vi "ctet_smu_User Main.vi"() -> ()   [LabVIEW 2019, in "ctet_smu User Library.lvlib"]
uses:
  ctet_smu User Library.lvlib
  Servers/ctet_smu/ctet_smu Class/typeDefs/Server State Data.ctl
  Types/ctet_smu.ctl
  Servers/ctet_smu/ctet_smu Class/RPC Messages/measurementservice_SMUConfigResponse/measurementservice_SMUConfigResponse_Data.ctl
  Servers/ctet_smu/ctet_smu Class/RPC Messages/measurementservice_ErrorOut/measurementservice_ErrorOut_Data.ctl
  Servers/ctet_smu/ctet_smu Class/ctet_smu.lvclass/ctet_smu.ctl
  Servers/ctet_smu/ctet_smu Class/ctet_smu.lvclass
panel:
  out "error out":errorcluster
  in  "error in (no error)":errorcluster
  in  "Stop":bool
  in  "Server Address":string="0.0.0.0:50052"
  in  "Server Certificate File (.crt)":path
  in  "Server Key File (.key)":path
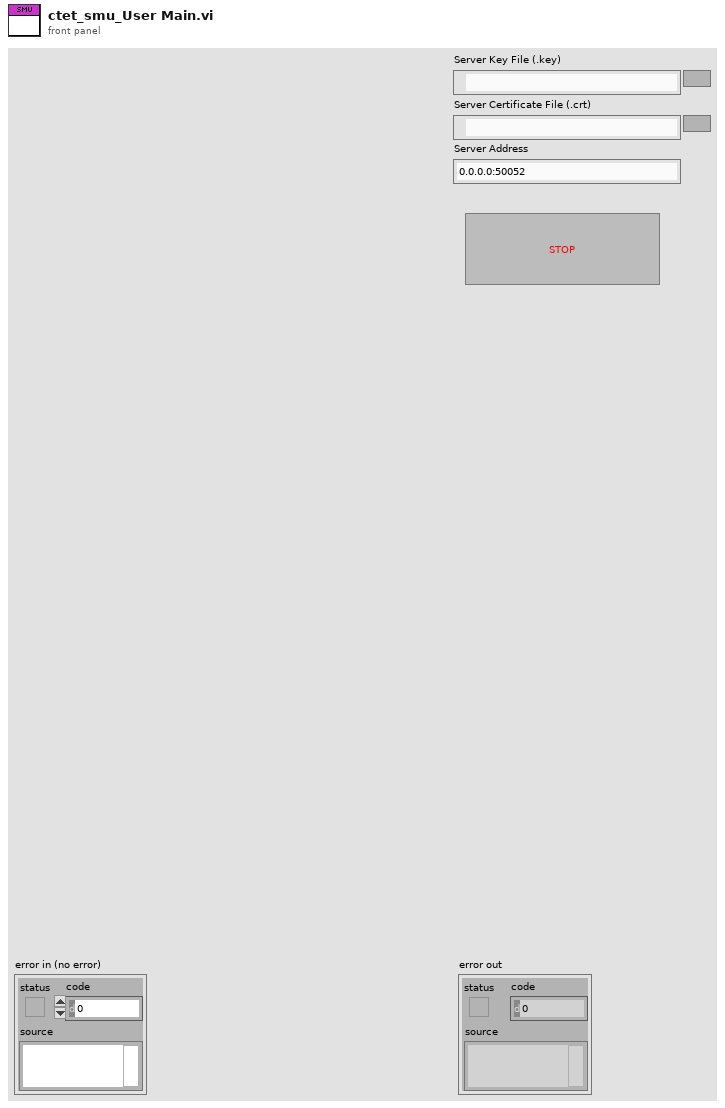
[diagram p1: front panel]
types:
  T1 = typedef "ctet_smu User Library.lvlib/ctet_smu.ctl" = cluster{"SMUSession":refnum<k15>, "measurementservice_SMUConfigResponse_Data":T2}
  T2 = typedef "ctet_smu.lvlib/ctet_smu.lvclass/measurementservice_SMUConfigResponse_Data.ctl" = cluster{"SMUChannels":string, "SMUSourceMode":i64, "SMUOutputFunction":i64, "SMUSourceTransientResponse":i64, "SMUCurrent":dbl, "SMUCurrentLevelRange":dbl, "SMUMeasurementSense":i64, "SMUApertureTimeUnit":i64, "SMUMeasurementApertureTime":dbl, "SMUSourceAdvancedSourceDelay":dbl, "SMUVoltage":dbl, "SMUMeasurementAdvancedDCNoiseRejection":i64, "error":T3}
  T3 = typedef "ctet_smu.lvlib/ctet_smu.lvclass/measurementservice_ErrorOut_Data.ctl" = cluster{"errCode":i64, "errMessage":string}
  T4 = typedef "ctet_smu.lvlib/ctet_smu.lvclass/Server State Data.ctl" = cluster{"Data":string}
  T5 = typedef "ctet_smu.lvlib/ctet_smu.lvclass/Server gRPC UEs.ctl" = cluster{"Invoke gRPC UE":refnum<user-event>, "Query gRPC UE":refnum<user-event>, "Register gRPC UE":refnum<user-event>, "OpenSMUSession gRPC UE":refnum<user-event>, "ConfigureSMU gRPC UE":refnum<user-event>, "EnableSMUOutput gRPC UE":refnum<user-event>, "DisableSMUOutput gRPC UE":refnum<user-event>, "PerformSMUCurrentMeasurement gRPC UE":refnum<user-event>, "CloseSMUSession gRPC UE":refnum<user-event>, "SelfCalibrateSMU gRPC UE":refnum<user-event>, "ResetSMU gRPC UE":refnum<user-event>, "GetSMULastExtCalInfo gRPC UE":refnum<user-event>, "GetSMULastSelfCalInfo gRPC UE":refnum<user-event>}
  T6 = typedef "ctet_smu.lvlib/gprc-lvsupport.lvlib/grpcId.ctl" = u64
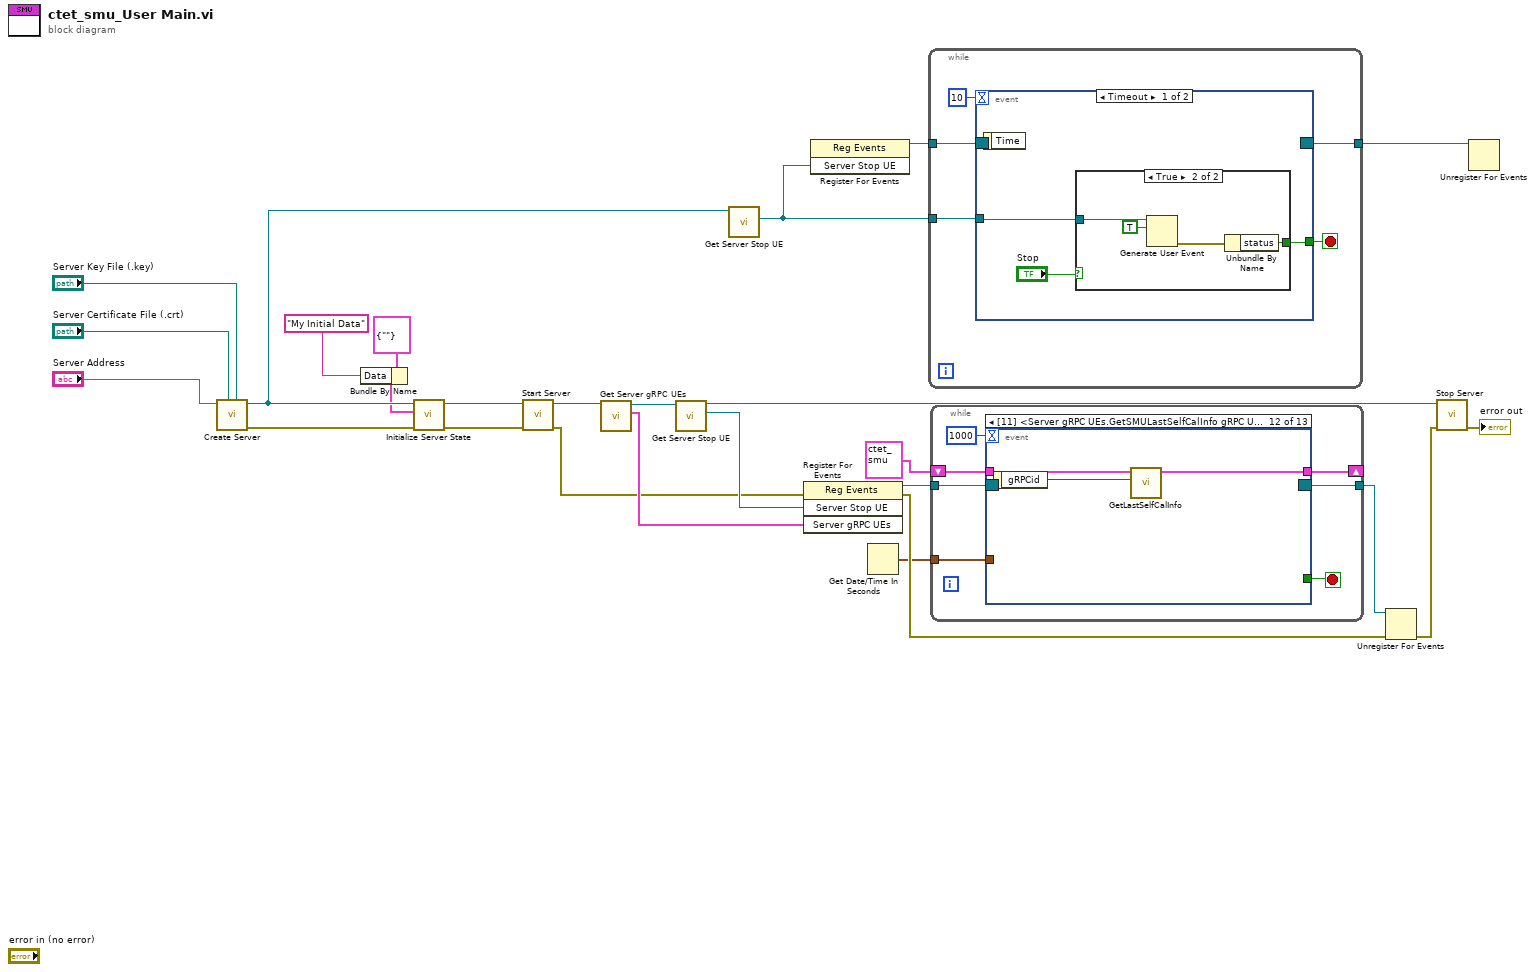
[diagram p0: block diagram]
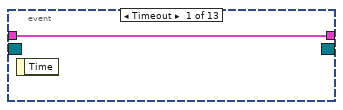
[diagram p2: hidden frame]
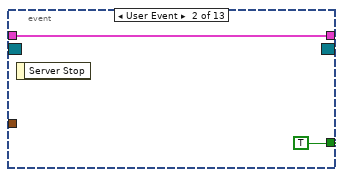
[diagram p3: hidden frame]
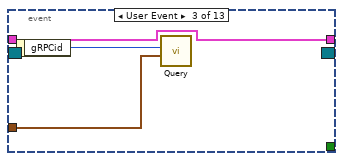
[diagram p4: hidden frame]
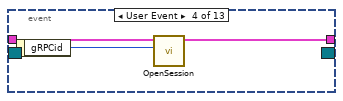
[diagram p5: hidden frame]
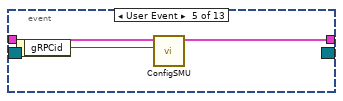
[diagram p6: hidden frame]
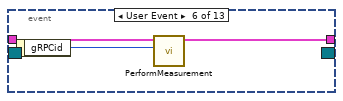
[diagram p7: hidden frame]
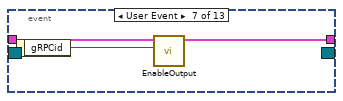
[diagram p8: hidden frame]
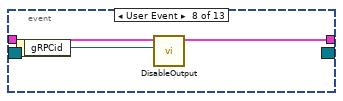
[diagram p9: hidden frame]
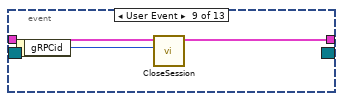
[diagram p10: hidden frame]
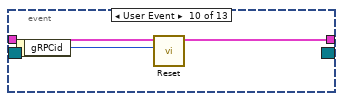
[diagram p11: hidden frame]
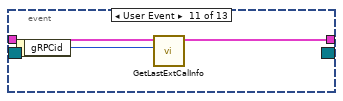
[diagram p12: hidden frame]
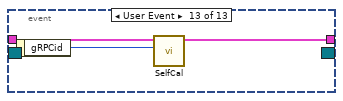
[diagram p13: hidden frame]
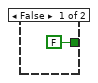
[diagram p14: hidden frame]
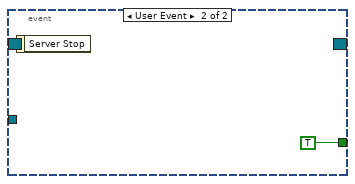
[diagram p15: hidden frame]
diagram:
  n1 = call "Create Server.vi"("Server Key File (.key)"="Server Key File (.key)", "Server Certificate File (.crt)"="Server Certificate File (.crt)", "Server Address"="Server Address") -> ("error out"=w20:errorcluster, "gRPC Server out"=w17:refnum<class "ctet_smu.lvclass">)  [unwired: 7 in]
  n2 = Bundle By Name(cluster=T4 {"Data"=""} ("Initial State"), "Data"="My Initial Data") -> (w15:T4)
  n3 = call "Initialize Server State.vi"("error in (no error)"=w20, "Initial State"=w15, "gRPC Server in"=w17) -> ("error out"=w19:errorcluster, "gRPC Server out"=w18:refnum<class "ctet_smu.lvclass">)  [unwired: 7 in]
  n4 = call "Start Server.vi"("error in (no error)"=w19, "gRPC Server in"=w18) -> ("error out"=w7:errorcluster, "gRPC Server out"=w8:refnum<class "ctet_smu.lvclass">)  [unwired: 8 in]
  n5 = call "Get Server gRPC UEs.vi"("OOP Server in"=w8) -> ("Server gRPC UEs"=w11:T5, "OOP Server out"=w13:refnum<class "ctet_smu.lvclass">)  [unwired: 9 in]
  n6 = call "Get Server Stop UE.vi"("OOP Server in"=w13) -> ("Server Stop UE"=w12:refnum<user-event>, "OOP Server out"=w5:refnum<class "ctet_smu.lvclass">)  [unwired: 9 in]
  n7 = call "Get Server Stop UE.vi"("OOP Server in"=w17) -> ("Server Stop UE"=w21:refnum<user-event>)  [unwired: 9 in, 1 out]
  n8 = register-events(error in=w7, w12, w11) -> (reference out=w10:refnum<event-registration>, error out=w6:errorcluster)  [unwired: 1 in]
  n9 = register-events(w21) -> (reference out=w23:refnum<event-registration>)  [unwired: 2 in, 1 out]
  n10 = Get Date/Time In Seconds() -> (seconds since 1Jan1904=w2:timestamp)
  n11 = while {
    tunnel: w21 -> [w31]
    tunnel: w23 -> [w30]
    tunnel: [w28] -> w22
    stop <- w29 stop-if-true
    n12 = event shown="[0] Timeout" {
      selector: w30 -> [_ _]
      dyn-events: [_ _] -> w28
      timeout: 10 -> [_ _]
      tunnel: w31 -> [w34 _]
      tunnel: [w33 TRUE] -> w29
      event Timeout {
        n13 = event-data() -> ()  [unwired: 1 in, 1 out]
        n14 = case shown="True" "Stop" {
          tunnel: w34 -> [_ w37]
          tunnel: [FALSE ("status") w36] -> w33
          frame False {
          }
          frame True {
            n15 = Generate User Event(user event=w37, event data cluster=TRUE ("event data")) -> (error out=w38:errorcluster)  [unwired: 2 in, 1 out]
            n16 = Unbundle By Name(w38) -> ("status"=w36:bool)
          }
        }
      }
      event User Event {
        n17 = event-data() -> ()  [unwired: 1 in, 1 out]
      }
    }
  }
  n18 = while {
    tunnel: w10 -> [w47]
    tunnel: [w45] -> w9
    tunnel: w2 -> [w43]
    shift-right: [w41] -> _
    shift-left: T1 {"SMUSession"="", "measurementservice_SMUConfigResponse_Data"={"SMUChannels"="", "SMUSourceMode"=0, "SMUOutputFunction"=0, "SMUSourceTransientResponse"=0, "SMUCurrent"=0.0, "SMUCurrentLevelRange"=0.0, "SMUMeasurementSense"=0, "SMUApertureTimeUnit"=0, "SMUMeasurementApertureTime"=0.0, "SMUSourceAdvancedSourceDelay"=0.0, "SMUVoltage"=0.0, "SMUMeasurementAdvancedDCNoiseRejection"=0, "error"={"errCode"=0, "errMessage"=""}}} ("ctet_smu") -> [w42]
    stop <- w46 stop-if-true
    n19 = event "RPC Methods Event Structure" shown="[11] <Server gRPC UEs.GetSMULastSelfCalInfo gRPC UE>: User Event" {
      selector: w47 -> [_ _ _ _ _ _ _ _ _ _ _ _ _]
      dyn-events: [_ _ _ _ _ _ _ _ _ _ _ _ _] -> w45
      timeout: 1000 -> [_ _ _ _ _ _ _ _ _ _ _ _ _]
      tunnel: [_ TRUE _ _ _ _ _ _ _ _ _ _ _] -> w46
      tunnel: w43 -> [_ _ w53 _ _ _ _ _ _ _ _ _ _]
      tunnel: w42 -> [w48 w49 w51 w55 w58 w61 w64 w67 w70 w73 w76 w79 w82]
      tunnel: [w48 w49 w51 w54 w57 w60 w63 w66 w69 w72 w75 w78 w81] -> w41
      event Timeout {
        n20 = event-data() -> ()  [unwired: 1 in, 1 out]
      }
      event User Event {
        n21 = event-data() -> ()  [unwired: 1 in, 1 out]
      }
      event User Event {
        n22 = event-data() -> ("gRPCid"=w52:T6)  [unwired: 1 in]
        n23 = call "Query.vi"("current time"=w53, "gRPCid"=w52) -> ()  [unwired: 9 in, 1 out]
      }
      event User Event {
        n24 = event-data() -> ("gRPCid"=w56:T6)  [unwired: 1 in]
        n25 = call "OpenSession.vi"("gRPCid"=w56, "ctet_smu"=w55) -> ("ctet_smu out"=w54:T1)  [unwired: 8 in, 1 out]
      }
      event User Event {
        n26 = event-data() -> ("gRPCid"=w59:T6)  [unwired: 1 in]
        n27 = call "ConfigSMU.vi"("gRPCid"=w59, "ctet_smu"=w58) -> ("ctet_smu out"=w57:T1)  [unwired: 8 in, 1 out]
      }
      event User Event {
        n28 = event-data() -> ("gRPCid"=w62:T6)  [unwired: 1 in]
        n29 = call "PerformMeasurement.vi"("gRPCid"=w62, "ctet_smu"=w61) -> ("ctet_smu out"=w60:T1)  [unwired: 8 in, 1 out]
      }
      event User Event {
        n30 = event-data() -> ("gRPCid"=w65:T6)  [unwired: 1 in]
        n31 = call "EnableOutput.vi"("gRPCid"=w65, "ctet_smu"=w64) -> ("ctet_smu out"=w63:T1)  [unwired: 8 in, 1 out]
      }
      event User Event {
        n32 = event-data() -> ("gRPCid"=w68:T6)  [unwired: 1 in]
        n33 = call "DisableOutput.vi"("gRPCid"=w68, "ctet_smu"=w67) -> ("ctet_smu out"=w66:T1)  [unwired: 8 in, 1 out]
      }
      event User Event {
        n34 = event-data() -> ("gRPCid"=w71:T6)  [unwired: 1 in]
        n35 = call "CloseSession.vi"("gRPCid"=w71, "ctet_smu"=w70) -> ("ctet_smu out"=w69:T1)  [unwired: 8 in, 1 out]
      }
      event User Event {
        n36 = event-data() -> ("gRPCid"=w74:T6)  [unwired: 1 in]
        n37 = call "Reset.vi"("gRPCid"=w74, "ctet_smu"=w73) -> ("ctet_smu out"=w72:T1)  [unwired: 8 in, 1 out]
      }
      event User Event {
        n38 = event-data() -> ("gRPCid"=w77:T6)  [unwired: 1 in]
        n39 = call "GetLastExtCalInfo.vi"("gRPCid"=w77, "ctet_smu"=w76) -> ("ctet_smu out"=w75:T1)  [unwired: 8 in, 1 out]
      }
      event User Event {
        n40 = event-data() -> ("gRPCid"=w80:T6)  [unwired: 1 in]
        n41 = call "GetLastSelfCalInfo.vi"("gRPCid"=w80, "ctet_smu"=w79) -> ("ctet_smu out"=w78:T1)  [unwired: 8 in, 1 out]
      }
      event User Event {
        n42 = event-data() -> ("gRPCid"=w83:T6)  [unwired: 1 in]
        n43 = call "SelfCal.vi"("gRPCid"=w83, "ctet_smu"=w82) -> ("ctet_smu out"=w81:T1)  [unwired: 8 in, 1 out]
      }
    }
  }
  n44 = Unregister For Events(event registration refnum=w9, error in=w6) -> (error out=w4:errorcluster)
  n45 = call "Stop Server.vi"("error in (no error)"=w4, "gRPC Server in"=w5) -> ("error out"=→"error out":errorcluster)  [unwired: 9 in]
  n46 = Unregister For Events(event registration refnum=w22) -> ()  [unwired: 1 in, 1 out]
